vi "Translation3d_ToTranslation2d.vi"(11 "In Translation3d":T2 {"Z" format="%14.3f"; "Y" format="%14.3f"; "X" format="%14.3f"}) -> (3 "Translation2d":T1 {"Y" format="%14.3f"; "X" format="%14.3f"})   [LabVIEW 2019, in "Trajectory_Library.lvlib"]
doc: "Returns a Translation2d representing this Translation3d projected into the X-Y plane.\n\nParameters\n - IN Translation3d - This Translation3d data structure\n\nReturns:\n - out Translation2d -- A Translation2d representing this Translation3d projected into the X-Y"
uses:
  Trajectory_Library.lvlib
  TypeDef/TRANSLATION3D.ctl
  TypeDef/TRANSLATION2D.ctl
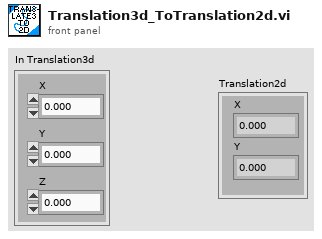
[diagram p1: front panel]
types:
  T1 = typedef "Trajectory_Library.lvlib/TRANSLATION2D.ctl" = cluster{"X":dbl, "Y":dbl}
  T2 = typedef "Trajectory_Library.lvlib/TRANSLATION3D.ctl" = cluster{"X":dbl, "Y":dbl, "Z":dbl}
  T3 = typedef "WPILib_Math.lvlib/TRANSLATION2D.ctl" = cluster{"X":dbl, "Y":dbl}
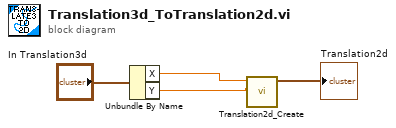
[diagram p0: block diagram]
diagram:
  n1 = Unbundle By Name("In Translation3d") -> ("X"=w2:dbl, "Y"=w1:dbl)
  n2 = call "Translation2d_Create.vi"("Y"=w1, "X"=w2) -> ("TRANSLATION"=→"Translation2d":T3)  [unwired: 9 in]
